vi "subDAQ_GetMoviePoint.vi"(5 "Recorde Table Refnum":refnum<vi>, 7 "Snap Number Refnum":refnum<vi>, 8 "Movie Point Y Arr Refnum":refnum<vi>, 9 "Movie Point X Arr Refnum":refnum<vi>, 10 "Snap Number Counting":dbl=2.0, 11 "Stage Status":T1={" Current Position"=[-1.0, -12.0, 0.0], "Number of Axis"=3, "ILSID"=1}) -> (1 "Snap/Movie Point cluster":cluster{"Snap Y":dbl[], "Snap X":dbl[]}, 2 "Movie Point  Y Array":dbl[](array[numeric]), 3 "Movie Point  X Array":dbl[](array[numeric]))   [LabVIEW 2015]
panel:
  # "X"
  # "Y"
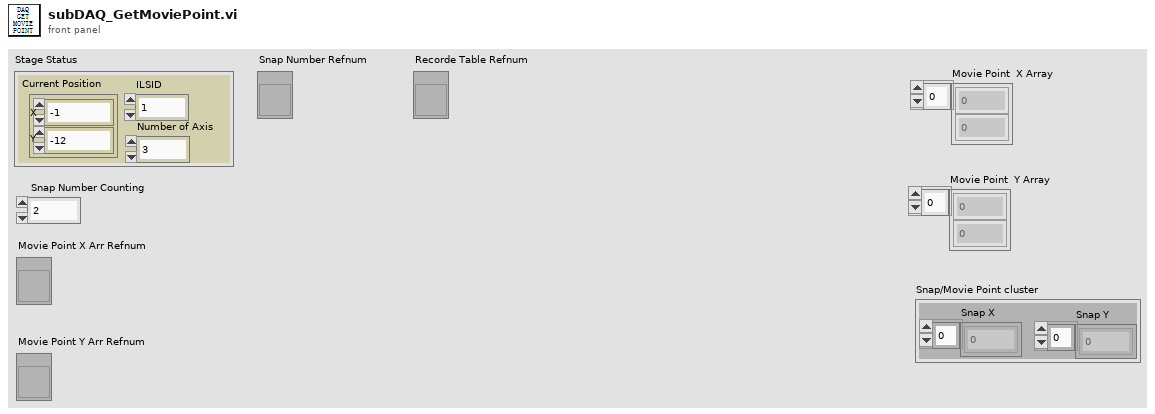
[diagram p1: front panel]
types:
  T1 = cluster{" Current Position":dbl[], "Number of Axis":i32, "ILSID":i32}
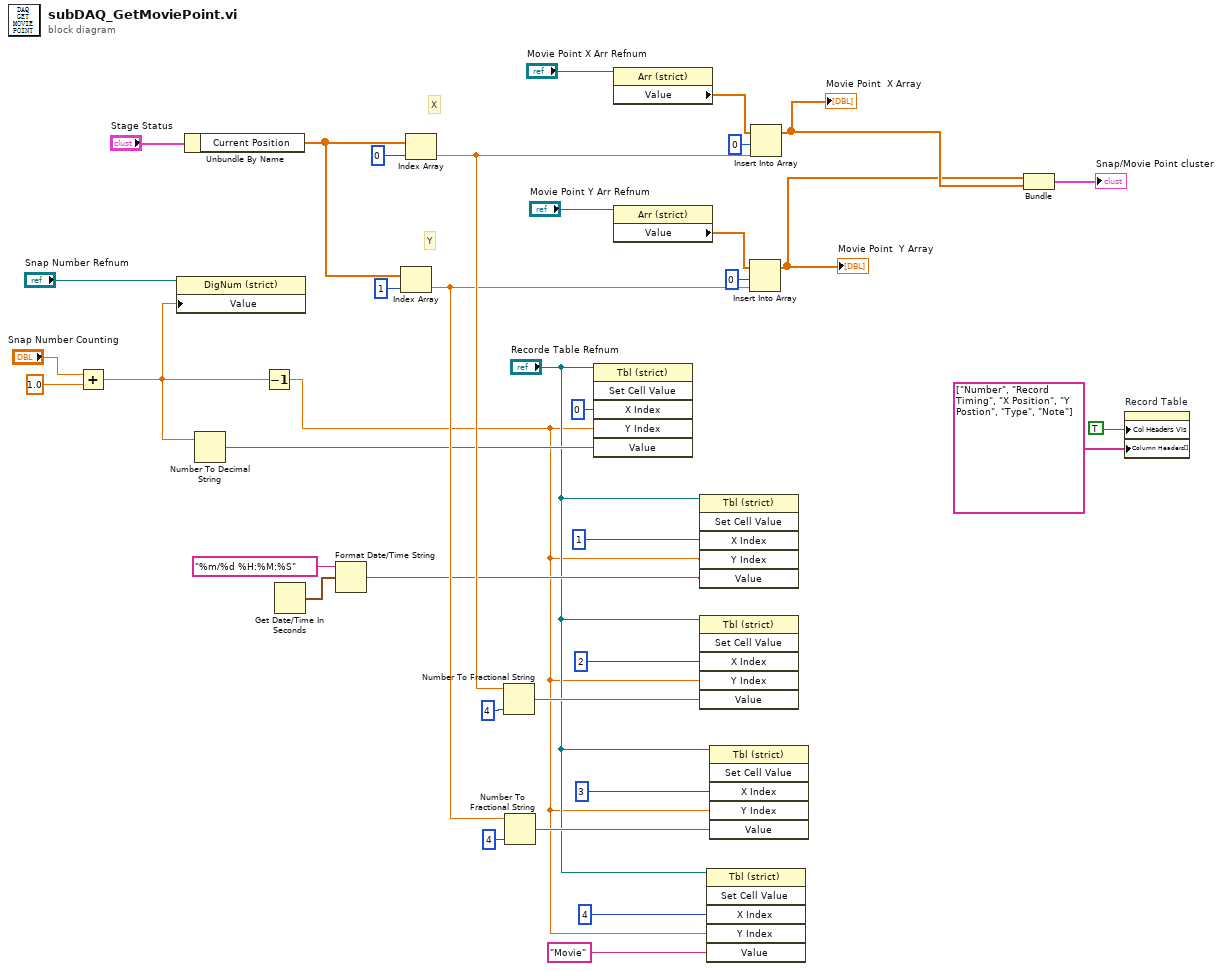
[diagram p0: block diagram]
diagram:
  # "Y"
  # "X"
  n1 = Add(x="Snap Number Counting", y=1.0) -> (x+y=w2:dbl)
  n2 = property class="DigNum (strict)"(reference="Snap Number Refnum", "Value"=w2) -> ()  [unwired: 1 in, 2 out]
  n3 = Unbundle By Name("Stage Status") -> ("Current Position"=w34:dbl[])
  n4 = Number To Decimal String(number=w2) -> (decimal integer string=w14:string)  [unwired: 1 in]
  n5 = Decrement(x=w2) -> (x-1=w1:dbl)
  n6 = Get Date/Time In Seconds() -> (seconds since 1Jan1904=w22:timestamp)
  n7 = Format Date/Time String(time format string (%c)="%m/%d %H:%M:%S", seconds (now)=w22) -> (date/time string=w12:string)  [unwired: 1 in]
  n8 = Index Array(array=w34, index=1) -> (element=w17:dbl)
  n9 = Index Array(array=w34, index=0) -> (element=w19:dbl)
  n10 = Number To Fractional String(number=w19, precision (6)=i16 4) -> (F-format string=w10:string)  [unwired: 2 in]
  n11 = Number To Fractional String(number=w17, precision (6)=i16 4) -> (F-format string=w8:string)  [unwired: 2 in]
  n12 = invoke class="Tbl (strict)" method="Set Cell Value"(reference="Recorde Table Refnum", "X Index"=0, "Y Index"=w1, "Value"=w14) -> ()  [unwired: 2 in, 6 out]
  n13 = property class="Arr (strict)"(reference="Movie Point X Arr Refnum") -> ("Value"=w27:dbl[])  [unwired: 1 in, 2 out]
  n14 = property class="Arr (strict)"(reference="Movie Point Y Arr Refnum") -> ("Value"=w25:dbl[])  [unwired: 1 in, 2 out]
  n15 = invoke class="Tbl (strict)" method="Set Cell Value"(reference="Recorde Table Refnum", "X Index"=1, "Y Index"=w1, "Value"=w12) -> ()  [unwired: 2 in, 6 out]
  n16 = invoke class="Tbl (strict)" method="Set Cell Value"(reference="Recorde Table Refnum", "X Index"=2, "Y Index"=w1, "Value"=w10) -> ()  [unwired: 2 in, 6 out]
  n17 = invoke class="Tbl (strict)" method="Set Cell Value"(reference="Recorde Table Refnum", "X Index"=4, "Y Index"=w1, "Value"="Movie") -> ()  [unwired: 2 in, 6 out]
  n18 = invoke class="Tbl (strict)" method="Set Cell Value"(reference="Recorde Table Refnum", "X Index"=3, "Y Index"=w1, "Value"=w8) -> ()  [unwired: 2 in, 6 out]
  n19 = Insert Into Array(array=w25, index=0, new element=w17) -> (w29:dbl[])
  "Movie Point  Y Array" <- w29
  n20 = Insert Into Array(array=w27, index=0, new element=w19) -> (w30:dbl[])
  "Movie Point  X Array" <- w30
  n21 = Bundle("Value"=w29, "Value"=w30) -> (→"Snap/Movie Point cluster":cluster{"Value":dbl[], "Value":dbl[]})  [unwired: 1 in]
  n22 = property on="Record Table" class="Tbl (strict)"("Col Headers Vis"=TRUE ("Visible Items:Column Headers Visible"), "Column Headers[]"=string[] ["Number", "Record Timing", "X Position", "Y Postion", "Type", "Note"] ("Column Header Strings[]")) -> ()  [unwired: 2 in, 2 out]
